vi "Write index_ptr.vi"(8 "error in (no error)":errorcluster, 10 "index_ptr":u64, 11 "KD Tree in":refnum<class "KD Tree.lvclass">) -> (0 "error out":errorcluster, 3 "KD Tree out":refnum<class "KD Tree.lvclass">)   [LabVIEW 2020, in "KD Tree.lvlib" / "KD Tree.lvclass"]
uses:
  KD Tree.lvclass
  KD Tree.lvclass/KD Tree.ctl
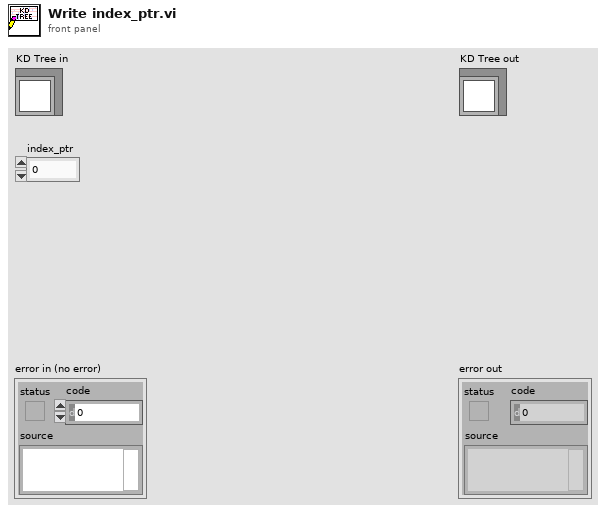
[diagram p1: front panel]
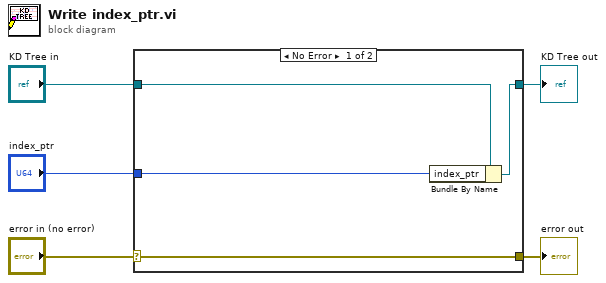
[diagram p0: block diagram]
diagram:
  n1 = case shown="No Error" "error in (no error)" {
    selector: "error in (no error)" -> [w9 w10]
    tunnel: [w9 w10] -> w4
    tunnel: [w7 w11] -> w2
    tunnel: "KD Tree in" -> [w8 w11]
    tunnel: "index_ptr" -> [w6 _]
    frame No Error {
      n2 = Bundle By Name(cluster=w8, "index_ptr"=w6) -> (w7:refnum<class "KD Tree.lvclass">)
    }
    frame Error {
    }
  }
  "error out" <- w4
  "KD Tree out" <- w2
